vi "Write CSV File.vi"() -> ()   [LabVIEW 2014]
uses:
  TEST_Control.ctl
  <vilib>/Utility/file.llb/Write To Spreadsheet File (string).vi
  <vilib>/Utility/file.llb/Write To Spreadsheet File (DBL).vi
panel:
  in  "Stop All":bool
  in  "stop":bool
  in  "Values to Write":i32=20
  in  "File String Template":string
  # "Generate Data"
  # "Write Header"
  # "Write Channel Names"
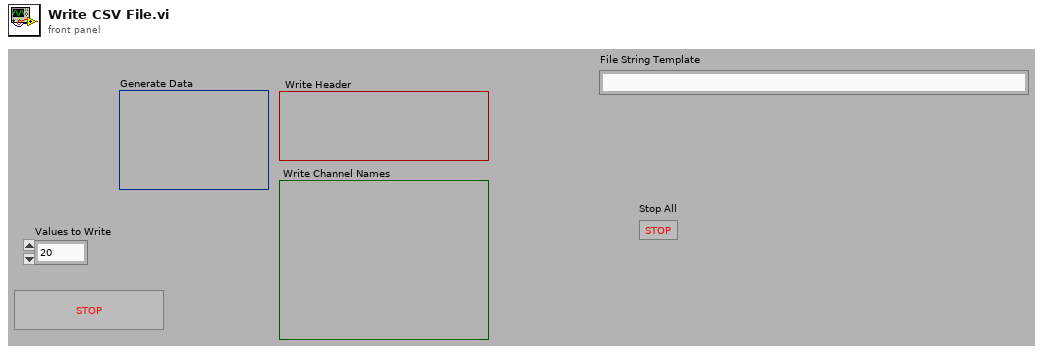
[diagram p1: front panel]
types:
  T1 = typedef "TEST_Control.ctl" = enum16{"Shutdown", "Init", "Write "}
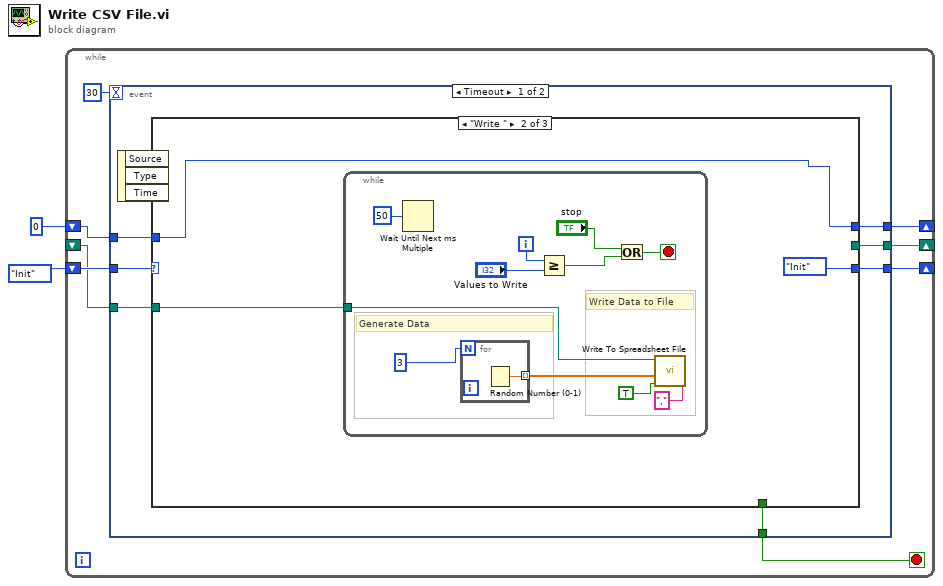
[diagram p0: block diagram]
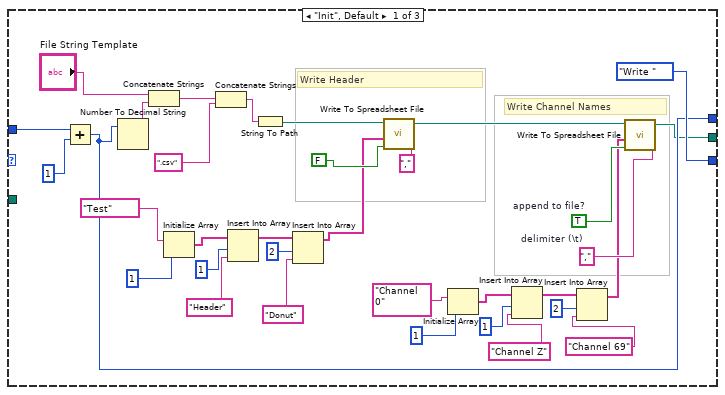
[diagram p2: hidden frame]
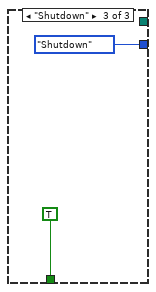
[diagram p3: hidden frame]
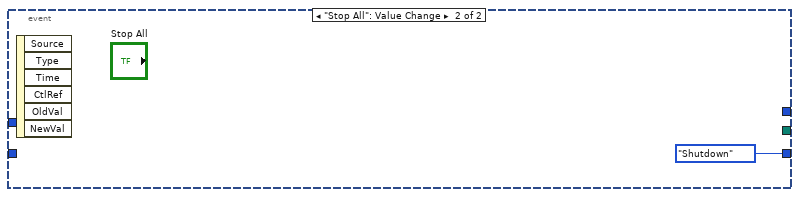
[diagram p4: hidden frame]
diagram:
  n1 = while {
    shift-right: [w9] -> _
    shift-left: 0 -> [w10]
    shift-right: [w8] -> _
    shift-left: TEST_Control."Init" -> [w7]
    shift-right: [w4] -> _
    shift-left: _ -> [w3]
    stop <- w5 stop-if-true
    n2 = event shown="[0] Timeout" {
      selector: _ -> [_ _]
      dyn-events: _ -> [_ _]
      timeout: 30 -> [_ _]
      tunnel: w10 -> [w17 _]
      tunnel: [w16 _] -> w9
      tunnel: [w15 TEST_Control."Shutdown"] -> w8
      tunnel: w7 -> [w14 _]
      tunnel: [w13 _] -> w5
      tunnel: [w12 _] -> w4
      tunnel: w3 -> [w11 _]
      event Timeout {
        n3 = event-data() -> ()  [unwired: 1 in, 3 out]
        n4 = case shown="\"Write \"" w14 {
          tunnel: w17 -> [w47 w53 _]
          tunnel: [w28 w53 _] -> w16
          tunnel: [TEST_Control."Write " TEST_Control."Init" TEST_Control."Shutdown"] -> w15
          tunnel: [_ _ TRUE] -> w13
          tunnel: [w27 _ _] -> w12
          tunnel: w11 -> [_ w52 _]
          frame "Init", Default {
            w50 = TRUE  # append to file?
            w48 = ","  # delimiter (\t)
            # "Write Header"
            # "Write Channel Names"
            n5 = Add(x=w47, y=1 ("x+y")) -> (x+y=w28:i32)
            n6 = Number To Decimal String(number=w28) -> (decimal integer string=w45:string)  [unwired: 1 in]
            n7 = Concatenate Strings("File String Template", w45) -> (w41:string)
            n8 = Initialize Array("Test", 1 ("dimension size")) -> (w37:string[])
            n9 = Concatenate Strings(w41, ".csv" ("string")) -> (w42:string)
            n10 = Insert Into Array(array=w37, index=1, new element="Header") -> (w36:string[])
            n11 = String To Path(string=w42) -> (path=w44:path)
            n12 = Insert Into Array(array=w36, index=2, new element="Donut") -> (w29:string[])
            n13 = call-poly <vilib>:"Write To Spreadsheet File.vi"("delimiter (\\t)"="," ("delimiter (\\t)"), "append to file? (new file:F)"=FALSE, "1D data"=w29, "file path (dialog if empty)"=w44) -> ("new file path (Not A Path if cancelled)"=w49:path)  [unwired: 3 in, 1 out]
            n14 = Initialize Array("Channel 0", 1 ("dimension size")) -> (w26:string[])
            n15 = Insert Into Array(array=w26, index=1, new element="Channel Z") -> (w25:string[])
            n16 = Insert Into Array(array=w25, index=2, new element="Channel 69") -> (w20:string[])
            n17 = call-poly <vilib>:"Write To Spreadsheet File.vi"("delimiter (\\t)"=w48, "append to file? (new file:F)"=w50, "1D data"=w20, "file path (dialog if empty)"=w49) -> ("new file path (Not A Path if cancelled)"=w27:path)  [unwired: 3 in, 1 out]
          }
          frame "Write " {
            n18 = while {
              tunnel: w52 -> [w55]
              i -> [w62]
              stop <- w59 stop-if-true
              # "Write Data to File"
              # "Generate Data"
              n19 = Wait Until Next ms Multiple(millisecond multiple=u32 50) -> ()  [unwired: 1 out]
              n20 = for {
                N: 3 -> [_]
                tunnel: [w66] -> w58 mode=indexing
                n21 = Random Number (0-1)() -> (number: 0 to 1=w66:dbl)
              }
              n22 = Greater Or Equal?(x=w62, y="Values to Write") -> (x >= y?=w60:bool)
              n23 = Or(x="stop", y=w60) -> (x .or. y?=w59:bool)
              n24 = call-poly <vilib>:"Write To Spreadsheet File.vi"("delimiter (\\t)"="," ("delimiter (\\t)"), "append to file? (new file:F)"=TRUE, "1D data"=w58, "file path (dialog if empty)"=w55) -> ()  [unwired: 3 in, 2 out]
            }
          }
          frame "Shutdown" {
          }
        }
      }
      event "Stop All": Value Change {
        n25 = event-data() -> ()  [unwired: 1 in, 6 out]
      }
    }
  }
